vi "IO_LKG3000 GetCalcData.vi"() -> ()   [LabVIEW 2024]
uses:
  Keyance Demo Code/Keyence LK-G3000/Public/clusters/LKIF_FLOATVALUE.ctl
  Keyance Demo Code/Keyence LK-G3000/Public/enums/LKIF_FLOATRESULT.ctl
  Keyance Demo Code/Keyence LK-G3000/Keyence LK-G3000.lvlib
panel:
  out "CalcData2":T1 {"LKIF_FLOATRESULT" items=["VALID", "RANGEOVER_P", "RANGEOVER_N", "WAITING"]}
  out "CalcData1":T1 {"LKIF_FLOATRESULT" items=["VALID", "RANGEOVER_P", "RANGEOVER_N", "WAITING"]}
  out "Trend Graph":cluster{"Value":sgl, "Value":sgl}(graph)
  in  "Stop VI":bool
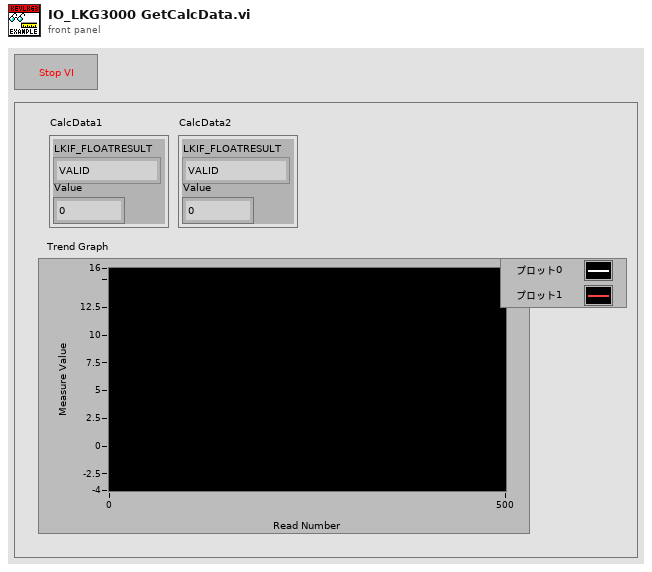
[diagram p1: front panel]
types:
  T1 = typedef "Keyence LK-G3000.lvlib/LKIF_FLOATVALUE.ctl" = cluster{"LKIF_FLOATRESULT":T2, "Value":sgl}
  T2 = typedef "Keyence LK-G3000.lvlib/LKIF_FLOATRESULT.ctl" = i32
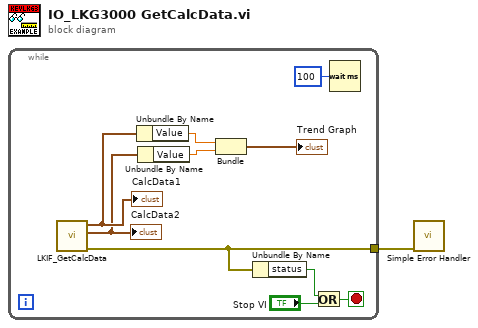
[diagram p0: block diagram]
diagram:
  n1 = while {
    tunnel: [w10] -> w1
    stop <- w11 stop-if-true
    n2 = call "LKIF_GetCalcData.vi"() -> ("error out"=w10:errorcluster, "CalcData2"=w5:T1, "CalcData1"=w6:T1)  [unwired: 9 in]
    "CalcData1" <- w6
    "CalcData2" <- w5
    n3 = Unbundle By Name(w6) -> ("Value"=w4:sgl)
    n4 = Unbundle By Name(w5) -> ("Value"=w3:sgl)
    n5 = Bundle("Value"=w4, "Value"=w3) -> (→"Trend Graph":cluster{"Value":sgl, "Value":sgl})  [unwired: 1 in]
    n6 = Unbundle By Name(w10) -> ("status"=w9:bool)
    n7 = Or(x=w9, y="Stop VI") -> (x .or. y?=w11:bool)
    n8 = Wait (ms)(milliseconds to wait=u32 100 ("ミリ秒待機時間")) -> ()  [unwired: 1 out]
  }
  n9 = call <vilib>:"Simple Error Handler.vi"("error in (no error)"=w1) -> ()  [unwired: 4 in, 5 out]
